vi "Get Number of Channels.vi"(11 "UI Data In":refnum<class "Settings UI.lvclass">) -> (0 "Channels Defined":bool, 1 "Num of Digital Channels":i32, 2 "Num of Analog Channels":i32, 3 "UI Data out":refnum<class "Settings UI.lvclass">)   [LabVIEW 2020, in "Output Sequencer.lvlib" / "Settings UI.lvclass"]
uses:
  Settings UI.lvclass
  Settings UI.lvclass/Settings UI.ctl
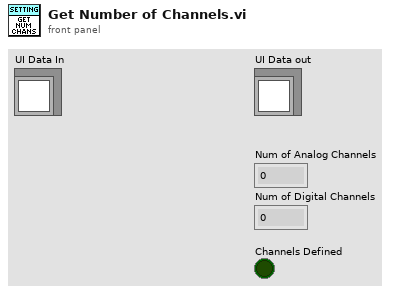
[diagram p1: front panel]
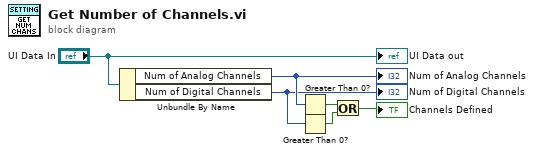
[diagram p0: block diagram]
diagram:
  n1 = Unbundle By Name("UI Data In") -> ("Num of Analog Channels"=w4:i32, "Num of Digital Channels"=w3:i32)
  "Num of Analog Channels" <- w4
  "Num of Digital Channels" <- w3
  n2 = Greater Than 0?(x=w4) -> (x > 0?=w6:bool)
  n3 = Greater Than 0?(x=w3) -> (x > 0?=w5:bool)
  n4 = Or(x=w6, y=w5) -> (x .or. y?=→"Channels Defined":bool)
  "UI Data out" <- "UI Data In"
